vi "zad3.vi"() -> ()   [LabVIEW 2025]
panel:
  out "RMS":dbl
  out "kw":dbl
  in  "input":dbl[](array[numeric])
  out "arytm":dbl
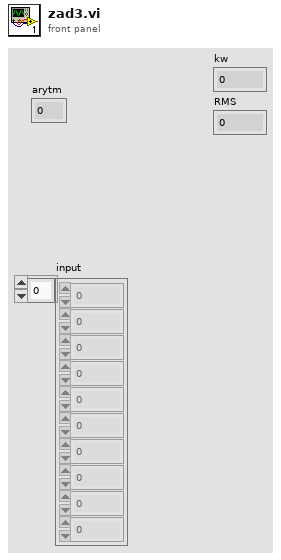
[diagram p1: front panel]
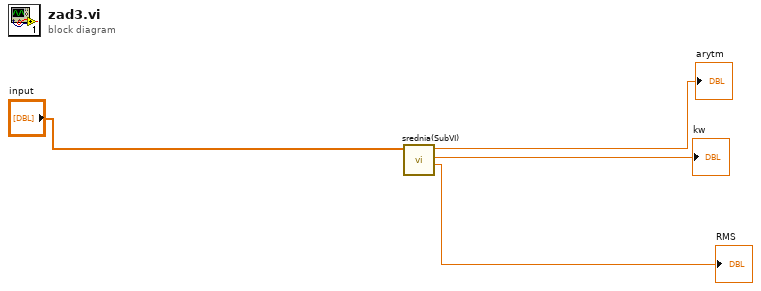
[diagram p0: block diagram]
diagram:
  n1 = call "srednia(SubVI).vi"("input"="input") -> ("RMS"=→"RMS":dbl, "kw"=→"kw":dbl, "arytm"=→"arytm":dbl)  [unwired: 8 in]
